vi "Init.vi"(8 "error in (no error)":errorcluster, 10 "Init Data":variant, 11 "CryoCoolerAVC in":refnum<class "CryoCoolerAVC.lvclass">) -> (0 "error out":errorcluster, 2 "Channel List":refnum<class "HK Item.lvclass">[](array[class]), 3 "CryoCoolerAVC out":refnum<class "CryoCoolerAVC.lvclass">)   [LabVIEW 2024, in "CryoCoolerAVC.lvclass"]
uses:
  CryoCoolerAVC.lvclass
  hk-channel-class/hk-channel-class/HK Item/HK Item.lvclass
  CryoCoolerAVC.lvclass/CryoCoolerAVC.ctl
  Cryo Cooler.lvclass
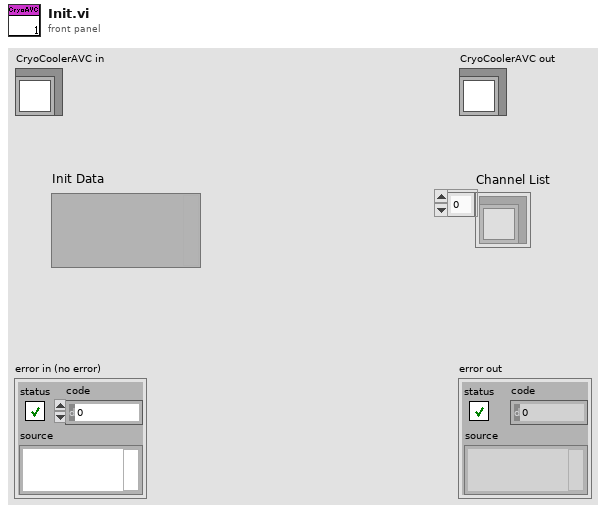
[diagram p1: front panel]
types:
  T1 = typedef "CryoCoolerAVC.lvclass/CryoCoolerAVC Settings.ctl" = cluster{"Cryo Addr":refnum<visa-resource-name>[]}
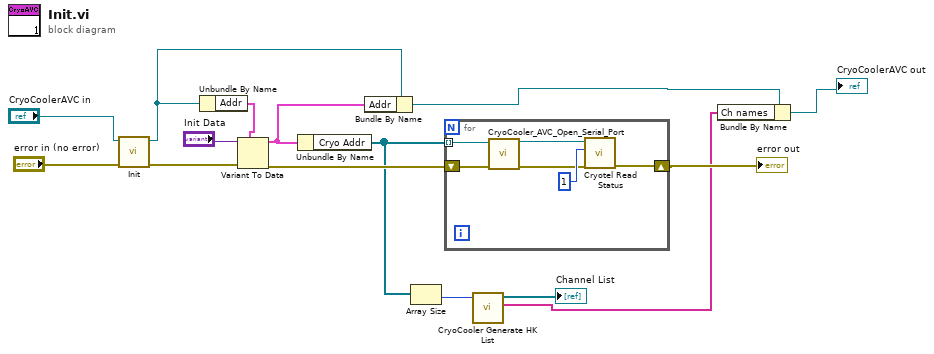
[diagram p0: block diagram]
diagram:
  n1 = call-parent "Init.vi"("error in (no error)"="error in (no error)", "Cryo Cooler in"="CryoCoolerAVC in") -> ("error out"=w13:errorcluster, "Cryo Cooler out"=w11:refnum<class "CryoCoolerAVC.lvclass">)  [unwired: 7 in, 1 out]
  n2 = Unbundle By Name(w11) -> ("Addr"=w10:T1)
  n3 = Variant To Data(error in=w13, type=w10, Variant="Init Data") -> (data=w9:T1, error out=w8:errorcluster)
  n4 = Unbundle By Name(w9) -> ("Cryo Addr"=w6:refnum<visa-resource-name>[])
  n5 = Bundle By Name(cluster=w11, "Addr"=w9) -> (w2:refnum<class "CryoCoolerAVC.lvclass">)
  n6 = Array Size(array=w6) -> (size(s)=w5:i32)
  n7 = for {
    tunnel: w6 -> [w20] mode=indexing
    shift-right: [w16] -> w7
    shift-left: w8 -> [w19]
    n8 = call "CryoCooler_AVC_Open_Serial_Port.vi"("error in (no error)"=w19, "VISA Resource (write)"=w20) -> ("error out"=w18:errorcluster, "VISA Resource out"=w17:refnum<visa-resource-name>)  [unwired: 8 in]
    n9 = call "Cryotel Read Status.vi"("error in"=w18, "Number of reads"=1, "VISA Resource (write)"=w17) -> ("error out"=w16:errorcluster)  [unwired: 6 in, 2 out]
  }
  "error out" <- w7
  n10 = call "CryoCooler Generate HK List.vi"("Num Cryos"=w5) -> ("Channel Names"=w3:string[], "Channel List"=→"Channel List":refnum<class "HK Item.lvclass">[])  [unwired: 9 in]
  n11 = Bundle By Name(cluster=w2, "Ch names"=w3) -> (→"CryoCoolerAVC out":refnum<class "CryoCoolerAVC.lvclass">)
